vi "create.orderbook.commands.for.testing.vi"(11 "OrderBook.Commands.in":T1[](array[typedef])=[{"type"=enum."AddOrder", "side"=66, "orderId "=48, "quantity"=20000, "symbol"=4702127773838221344, "price"=9050, "executed.qty"=0, "canceled.qty"=0, "remaining.qty"=0, "seconds"=0, "nanoseconds"=0}] {"symbol" format="%.0x"; "orderId" format="%.0x"; "side" format="%.0x"}) -> (3 "Words.Out":u64[](array[numeric])=[1, 66, 48, 20000, 4702127773838221344, 9050, 0, 0, 0, 0, 0, 0, 0, 0, 0, 0, 2, 66, 48, 0, 0, 9050, 200, 0, 0, 0, 0, 0, 0, 0, 0, 0, 5, 66, 48, 1400, 6076284164848492576, 9050, 0, 0, 0, 0, 0, 0, 0, 0, 0, 0] format="%.0x")   [LabVIEW 2022 SP3]
uses:
  fpga/common/orderbook.command.ctl
  fpga/common/orderbook.command.type.ctl
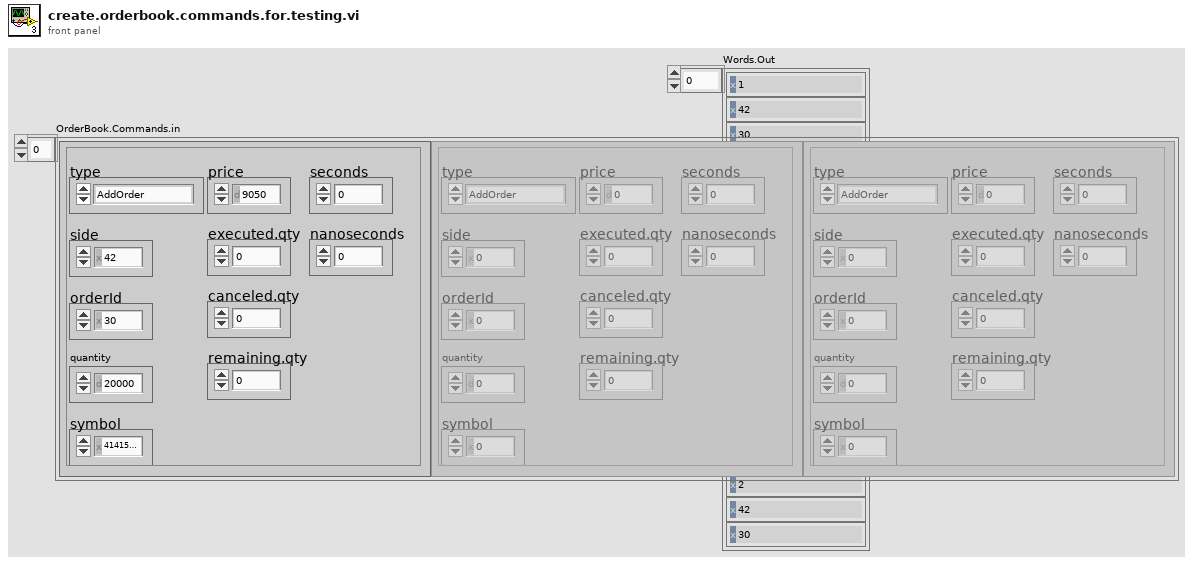
[diagram p1: front panel]
types:
  T1 = typedef "orderbook.command.ctl" = cluster{"type":T2, "side":u8, "orderId ":u64, "quantity":u32, "symbol":u64, "price":u64, "executed.qty":u32, "canceled.qty":u32, "remaining.qty":u32, "seconds":u64, "nanoseconds":u64}
  T2 = typedef "orderbook.command.type.ctl" = enum8{"Time", "AddOrder", "OrderExecuted", "OrderExecutedAtPrice", "ReduceSize", "ModifyOrder", "DeleteOrder", "Get.State", "Get.All.Orders", "Get.Top"}
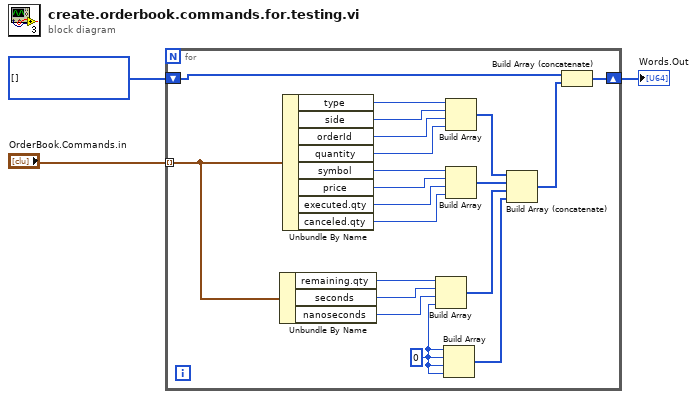
[diagram p0: block diagram]
diagram:
  n1 = for {
    tunnel: "OrderBook.Commands.in" -> [w23] mode=indexing
    shift-right: [w5] -> w1
    shift-left: u64[] [] -> [w7]
    w12 = u64 0 ("element")
    n2 = Unbundle By Name(w23) -> ("remaining.qty"=w14:u32, "seconds"=w13:u64, "nanoseconds"=w4:u64)
    n3 = Unbundle By Name(w23) -> ("type"=w22:T2, "side"=w21:u8, "orderId"=w20:u64, "quantity"=w19:u32, "symbol"=w18:u64, "price"=w17:u64, "executed.qty"=w16:u32, "canceled.qty"=w15:u32)
    n4 = Build Array(w14, w13, w4, w12) -> (w9:u64[])
    n5 = Build Array(w12, w12, w12, w12) -> (w8:u64[])
    n6 = Build Array(w22, w21, w20, w19) -> (w11:u64[])
    n7 = Build Array(w18, w17, w16, w15) -> (w10:u64[])
    n8 = Build Array (concatenate)(w11, w10, w9, w8) -> (w6:u64[])
    n9 = Build Array (concatenate)(w7, w6) -> (w5:u64[])
  }
  "Words.Out" <- w1
